vi "ScpiSendLog.vi"(8 "error in (no error)":errorcluster, 9 "Command":string, 10 "TCP port":u16=5025 min=1025 step=1, 11 "IP Address":string="localhost") -> (0 "error out":errorcluster)   [LabVIEW 2009]
doc: "Sends a SCPI command to an instrument, using TCP/IP.\nThen disconnects."
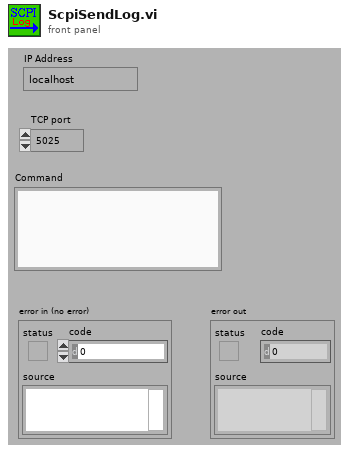
[diagram p1: front panel]
types:
  T1 = enum16{"Read_SCPI_Log_Status", "No_SCPI_Log", "Log_SCPI", "Reset"}
  T2 = enum16{"open", "replace", "create", "open or create", "replace or create", "replace or create with confirmation"}
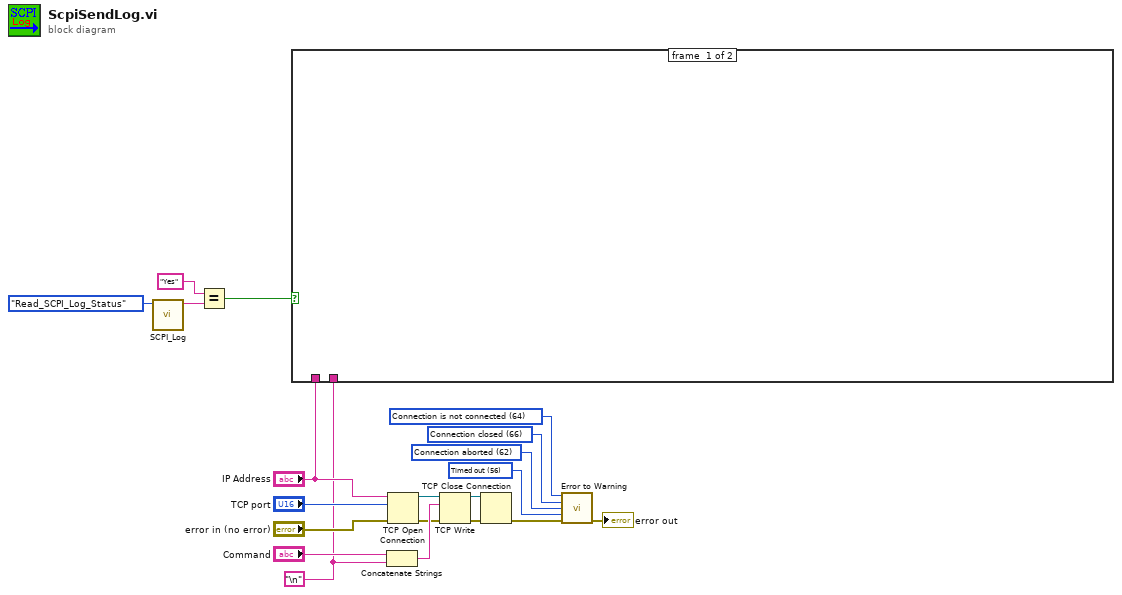
[diagram p0: block diagram]
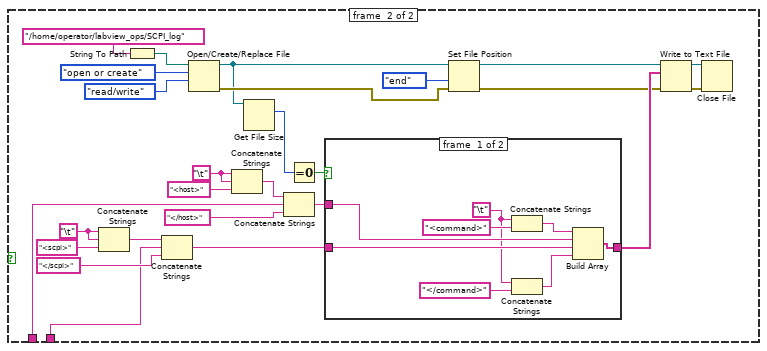
[diagram p2: hidden frame]
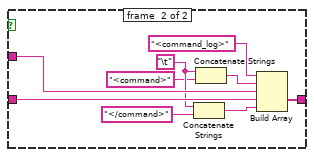
[diagram p3: hidden frame]
diagram:
  w10 = 56 items=["No Error", "Argument Error", "Memory Full", "Out of Zone", "End of File", "File Already Open", "Generic File IO Error", "File Not Found", "File Permission Error", "Disk Full", "Duplicate Path", "Too Many Files Open", "Not Enabled", "Resource File Not Found", "Cannot Add Resource", "Resource Not Found", "Image Not Found", "Image Memory Error", "Pen Does Not Exist", "Config Bad Type", "Config Token Not Found", "Config Parse Error", "Config Memory Error", "Bad External Code Format", "Bad External Code Offset", "External Code Not Present", "Null Window", "Destroy Window Mixup", "Null Menu", "Print Aborted", "Bad Print Record", "Print Driver Error", "Windows Error During Print", "Memory Error During Print", "Print Dialog Error", "Generic Print Error", "Invalid Device Refnum", "Device Not Found", "Device Parameter Error", "Device Unit Error", "Can't Open Device", "Device Call Aborted", "Generic Error", "Cancelled By User", "Object ID Too Low", "Object ID Too High", "Object Not In Heap", "Unknown Heap", "Bad DefProc ID", "DefProc Not In Table", "Message Out Of Range", "Null Method", "Unknown Message", "Manager Call Not Supported", "Bad address", "Connection In progress", "Timed out", "Connection is already in progress", "Network attribute not supported", "Network error", "Address in use", "System out of memory", "Connection aborted", "Connection refused", "Connection is not connected", "Connection is already connected", "Connection closed", "Initialize error (interapplication manager)", "Bad occurrence", "Wait on unbound occurrence handler", "Occurrence queue overflow", "Bad path", "Semaphore not signaled", "Unrecognized type (interapplication manager)"] ("1st Error to Convert")
  w1 = "\n"
  w15 = 62 items=["No Error", "Argument Error", "Memory Full", "Out of Zone", "End of File", "File Already Open", "Generic File IO Error", "File Not Found", "File Permission Error", "Disk Full", "Duplicate Path", "Too Many Files Open", "Not Enabled", "Resource File Not Found", "Cannot Add Resource", "Resource Not Found", "Image Not Found", "Image Memory Error", "Pen Does Not Exist", "Config Bad Type", "Config Token Not Found", "Config Parse Error", "Config Memory Error", "Bad External Code Format", "Bad External Code Offset", "External Code Not Present", "Null Window", "Destroy Window Mixup", "Null Menu", "Print Aborted", "Bad Print Record", "Print Driver Error", "Windows Error During Print", "Memory Error During Print", "Print Dialog Error", "Generic Print Error", "Invalid Device Refnum", "Device Not Found", "Device Parameter Error", "Device Unit Error", "Can't Open Device", "Device Call Aborted", "Generic Error", "Cancelled By User", "Object ID Too Low", "Object ID Too High", "Object Not In Heap", "Unknown Heap", "Bad DefProc ID", "DefProc Not In Table", "Message Out Of Range", "Null Method", "Unknown Message", "Manager Call Not Supported", "Bad address", "Connection In progress", "Connection timed out", "Connection is already in progress", "Network attribute not supported", "Network error", "Address in use", "System out of memory", "Connection aborted", "Connection refused", "Connection is not connected", "Connection is already connected", "Connection closed", "Initialize error (interapplication manager)", "Bad occurrence", "Wait on unbound occurrence handler", "Occurrence queue overflow", "Bad path", "Semaphore not signaled", "Unrecognized type (interapplication manager)"] ("1st Error to Convert")
  w16 = 66 items=["No Error", "Argument Error", "Memory Full", "Out of Zone", "End of File", "File Already Open", "Generic File IO Error", "File Not Found", "File Permission Error", "Disk Full", "Duplicate Path", "Too Many Files Open", "Not Enabled", "Resource File Not Found", "Cannot Add Resource", "Resource Not Found", "Image Not Found", "Image Memory Error", "Pen Does Not Exist", "Config Bad Type", "Config Token Not Found", "Config Parse Error", "Config Memory Error", "Bad External Code Format", "Bad External Code Offset", "External Code Not Present", "Null Window", "Destroy Window Mixup", "Null Menu", "Print Aborted", "Bad Print Record", "Print Driver Error", "Windows Error During Print", "Memory Error During Print", "Print Dialog Error", "Generic Print Error", "Invalid Device Refnum", "Device Not Found", "Device Parameter Error", "Device Unit Error", "Can't Open Device", "Device Call Aborted", "Generic Error", "Cancelled By User", "Object ID Too Low", "Object ID Too High", "Object Not In Heap", "Unknown Heap", "Bad DefProc ID", "DefProc Not In Table", "Message Out Of Range", "Null Method", "Unknown Message", "Manager Call Not Supported", "Bad address", "Connection In progress", "Connection timed out", "Connection is already in progress", "Network attribute not supported", "Network error", "Address in use", "System out of memory", "Connection aborted", "Connection refused", "Connection is not connected", "Connection is already connected", "Connection closed", "Initialize error (interapplication manager)", "Bad occurrence", "Wait on unbound occurrence handler", "Occurrence queue overflow", "Bad path", "Semaphore not signaled", "Unrecognized type (interapplication manager)"] ("1st Error to Convert")
  w17 = 64 items=["No Error", "Argument Error", "Memory Full", "Out of Zone", "End of File", "File Already Open", "Generic File IO Error", "File Not Found", "File Permission Error", "Disk Full", "Duplicate Path", "Too Many Files Open", "Not Enabled", "Resource File Not Found", "Cannot Add Resource", "Resource Not Found", "Image Not Found", "Image Memory Error", "Pen Does Not Exist", "Config Bad Type", "Config Token Not Found", "Config Parse Error", "Config Memory Error", "Bad External Code Format", "Bad External Code Offset", "External Code Not Present", "Null Window", "Destroy Window Mixup", "Null Menu", "Print Aborted", "Bad Print Record", "Print Driver Error", "Windows Error During Print", "Memory Error During Print", "Print Dialog Error", "Generic Print Error", "Invalid Device Refnum", "Device Not Found", "Device Parameter Error", "Device Unit Error", "Can't Open Device", "Device Call Aborted", "Generic Error", "Cancelled By User", "Object ID Too Low", "Object ID Too High", "Object Not In Heap", "Unknown Heap", "Bad DefProc ID", "DefProc Not In Table", "Message Out Of Range", "Null Method", "Unknown Message", "Manager Call Not Supported", "Bad address", "Connection In progress", "Connection timed out", "Connection is already in progress", "Network attribute not supported", "Network error", "Address in use", "System out of memory", "Connection aborted", "Connection refused", "Connection is not connected", "Connection is already connected", "Connection closed", "Initialize error (interapplication manager)", "Bad occurrence", "Wait on unbound occurrence handler", "Occurrence queue overflow", "Bad path", "Semaphore not signaled", "Unrecognized type (interapplication manager)"] ("1st Error to Convert")
  n1 = call "SCPI_Log.vi"("SCOP Log In"=T1."Read_SCPI_Log_Status") -> ("SCPI Log Out"=w5:string)  [unwired: 10 in]
  n2 = Equal?(x="Yes" ("SCPI Log Out"), y=w5) -> (x = y?=w4:bool)
  n3 = case shown="True" w4 {
    tunnel: "IP Address" -> [_ w32]
    tunnel: w1 -> [_ w21]
    frame #0 {
    }
    frame #1 {
      w25 = "\t"
      w24 = "\t"
      n4 = Concatenate Strings(w25, w25, "<scpi>") -> (w28:string)
      n5 = String To Path(string="/home/operator/labview_ops/SCPI_log" ("SCPI Log Out")) -> (path=w45:path)
      n6 = Concatenate Strings(w28, w21, "</scpi>") -> (w36:string)
      n7 = Open/Create/Replace File(file path (use dialog)=w45, operation (0:open)=T2."open or create", access (0:read/write)=enum16{"read/write", "read-only", "write-only"}."read/write") -> (refnum out=w35:refnum<file>, error out=w40:errorcluster)  [unwired: 3 in, 1 out]
      n8 = Concatenate Strings(w24, w24, "<host>") -> (w30:string)
      n9 = Get File Size(file=w35) -> (size (in bytes)=w33:i64)  [unwired: 1 in, 2 out]
      n10 = Concatenate Strings(w30, w32, "</host>") -> (w37:string)
      n11 = Equal To 0?(x=w33) -> (x = 0?=w34:bool)
      n12 = case shown="True" w34 {
        tunnel: w36 -> [w53 w63]
        tunnel: [w52 w62] -> w42
        tunnel: w37 -> [w54 w61]
        frame #0 {
          w47 = "\t"
          n13 = Concatenate Strings(w47, "<command>") -> (w50:string)
          n14 = Concatenate Strings(w47, "</command>") -> (w48:string)
          n15 = Build Array(w50, w54, w53, w48) -> (w52:string[])
        }
        frame #1 {
          w59 = "\t"
          n16 = Concatenate Strings(w59, "</command>") -> (w55:string)
          n17 = Concatenate Strings(w59, "<command>") -> (w56:string)
          n18 = Build Array("<command_log>", w56, w61, w63, w55) -> (w62:string[])
        }
      }
      n19 = Set File Position(refnum=w35, from (0:start)=enum16{"start", "end", "current"}."end", error in=w40) -> (refnum out=w43:refnum<file>, error out=w39:errorcluster)  [unwired: 1 in]
      n20 = Write to Text File(file (use dialog)=w43, text=w42, error in=w39) -> (refnum out=w23:refnum<file>, error out=w22:errorcluster)  [unwired: 1 in, 1 out]
      n21 = Close File(refnum=w23, error in=w22) -> ()  [unwired: 2 out]
    }
  }
  n22 = Concatenate Strings("Command", w1) -> (w13:string)
  n23 = TCP Open Connection(address="IP Address", remote port or service name="TCP port", error in (no error)="error in (no error)") -> (connection ID=w14:refnum<k5>, error out=w12:errorcluster)  [unwired: 2 in]
  n24 = TCP Write(connection ID=w14, data in=w13, error in (no error)=w12) -> (connection ID out=w9:refnum<k5>, error out=w8:errorcluster)  [unwired: 1 in, 1 out]
  n25 = TCP Close Connection(connection ID=w9, error in (no error)=w8) -> (error out=w19:errorcluster)  [unwired: 1 in, 1 out]
  n26 = call <vilib>:"Error to Warning.vi"("1st Error to Convert"=w17, "2nd Error to Convert"=w16, "3rd Error to Convert"=w15, "4th Error to Convert"=w10, "error in"=w19) -> ("warning out"=→"error out":errorcluster)  [unwired: 10 in]
